vi "Open File.vi"(8 "error in (no error)":errorcluster, 11 "TDMS in":refnum<class "TDMS.lvclass">) -> (0 "error out":errorcluster, 3 "TDMS out":refnum<class "TDMS.lvclass">)   [LabVIEW 2020, in "TDMS.lvclass"]
uses:
  TDMS.lvclass
  Abstrut Data/Abstruct Data Type.lvclass/Abstruct Data Type.ctl
  TDMS.lvclass/TDMS.ctl
  Abstrut Data/Accessors/Read File Path.vi
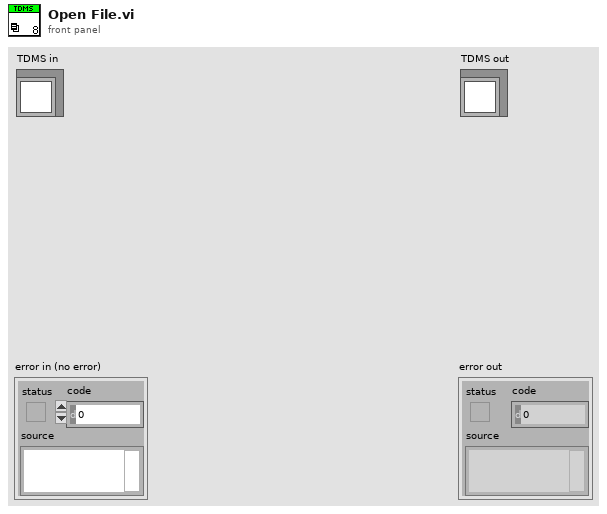
[diagram p1: front panel]
types:
  T1 = enum16{"open", "open or create", "create or replace", "create", "open (read-only)"}
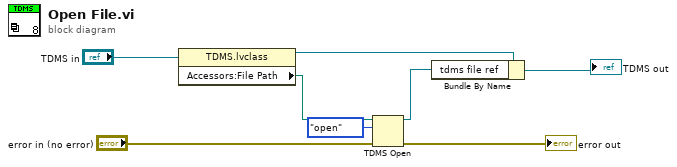
[diagram p0: block diagram]
diagram:
  n1 = property class="TDMS.lvclass"(reference="TDMS in") -> (reference out=w4:refnum<class "TDMS.lvclass">, "Accessors:File Path"=w7:path)  [unwired: 1 in, 1 out]
  n2 = TDMS Open(8:"error in (no error)", 10:T1."open" ("operation (0:open)"), 11:w7) -> (0:→"error out":errorcluster, 3:w3:refnum<k34>)  [unwired: 4 in]
  n3 = Bundle By Name(cluster=w4, "tdms file ref"=w3) -> (→"TDMS out":refnum<class "TDMS.lvclass">)
